vi "pessimize_error.vi"(8 "End transform offset":dbl[](array[numeric])=[0.0, 0.0, 0.0, 0.0, 0.0, 0.0] format="%#.3f", 9 "stop":refnum<vi>, 10 "Point selector":T7 {"Light number" min=0 max=5}, 11 "Override in":T6) -> ()   [LabVIEW 2013]
uses:
  calibration/point_selector.ctl
  ui_override_opts.ctl
  pessimize_objective_fun_info.ctl
  pressimize_state.ctl
  <vilib>/Utility/file.llb/Write To Spreadsheet File (DBL).vi
  <vilib>/Analysis/Matrix/Datatypes/RealMatrix.ctl
  <vilib>/Analysis/Matrix/NI_Matrix.lvlib
  <vilib>/gmath/NumericalOptimization/stopping criteria.ctl
  <vilib>/gmath/NI_Gmath.lvlib
panel:
  in  "Save":bool
  in  "Save file":path
  out "Trials":T1 format="%#_3p"
  in  "Random trials":i32=1
  out "Error vector":T1 format="%#_3p"
  out "Pose bias":T1 format="%#_3p"
  out "f(X) max":dbl format="%#_3p"
  in  "Random":bool
  in  "Last out":bool
  in  "GD gain":dbl=0.3
  in  "dX":T1=[[0.2, 1.0]]
  in  "Method":T2(ring)
  in  "Local stop":bool
  in  "Trace length":dbl=0.2
  in  "Moment":dbl=50.0
  in  "XY plots":cluster{"X":T3, "Y":T3}[](array[cluster])=[{"X"=enum."X", "Y"=enum."Y"}, {"X"=enum."X", "Y"=enum."Z"}, {"X"=enum."Rx", "Y"=enum."Ry"}, {"X"=enum."Rx", "Y"=enum."Rz"}]
  out "XY Graph":T4(graph)
  out "Function calls":i32 caption="Iterations"
  out "Function value":dbl[](graph)
  in  "Running":bool
  in  "Start point":T1 format="%#_3p"
  in  "Workspace bounds":T1=[[-15.0, -15.0, -15.0, -20.0, -20.0, -10.0], [15.0, 15.0, 15.0, 10.0, 20.0, 10.0]]
  in  "Optimization status":T1 format="%#_3p"
  in  "Scaling":T1=[[1.0, 0.2], [0.1, 1.0], [0.1, 0.1]]
  in  "Error criterion":enum16{"Translation", "Orientation", "Moment"}(ring)
  out "X at maximum":T1 format="%#_3p"
  in  "stopping criteria":T5={"function tolerance"=1.0, "parameter tolerance"=0.1, "max iterations"=100, "max function calls"=1000, "gradient tolerance"=0.01, "max time (sec)"=-1.0}
  # "--------XYZ--------      ---------Rxyz---------     --------eXYZ---------      --------eRxyz-------      eFun"
  # "XYZ"
  # "R"
  # "Min"
  # "Max"
  # "X"
  # "Y"
  # "Z"
  # "Rx"
  # "Ry"
  # "Rz"
  # "--------XYZ--------      ---------Rxyz---------     --------eXYZ---------      --------eRxyz-------      eFun       ------gradXYZ------      ------gradRxyz------"
  # "XYZ error"
  # "R error"
  # "Tolerance"
  # "Trans"
  # "Orient"
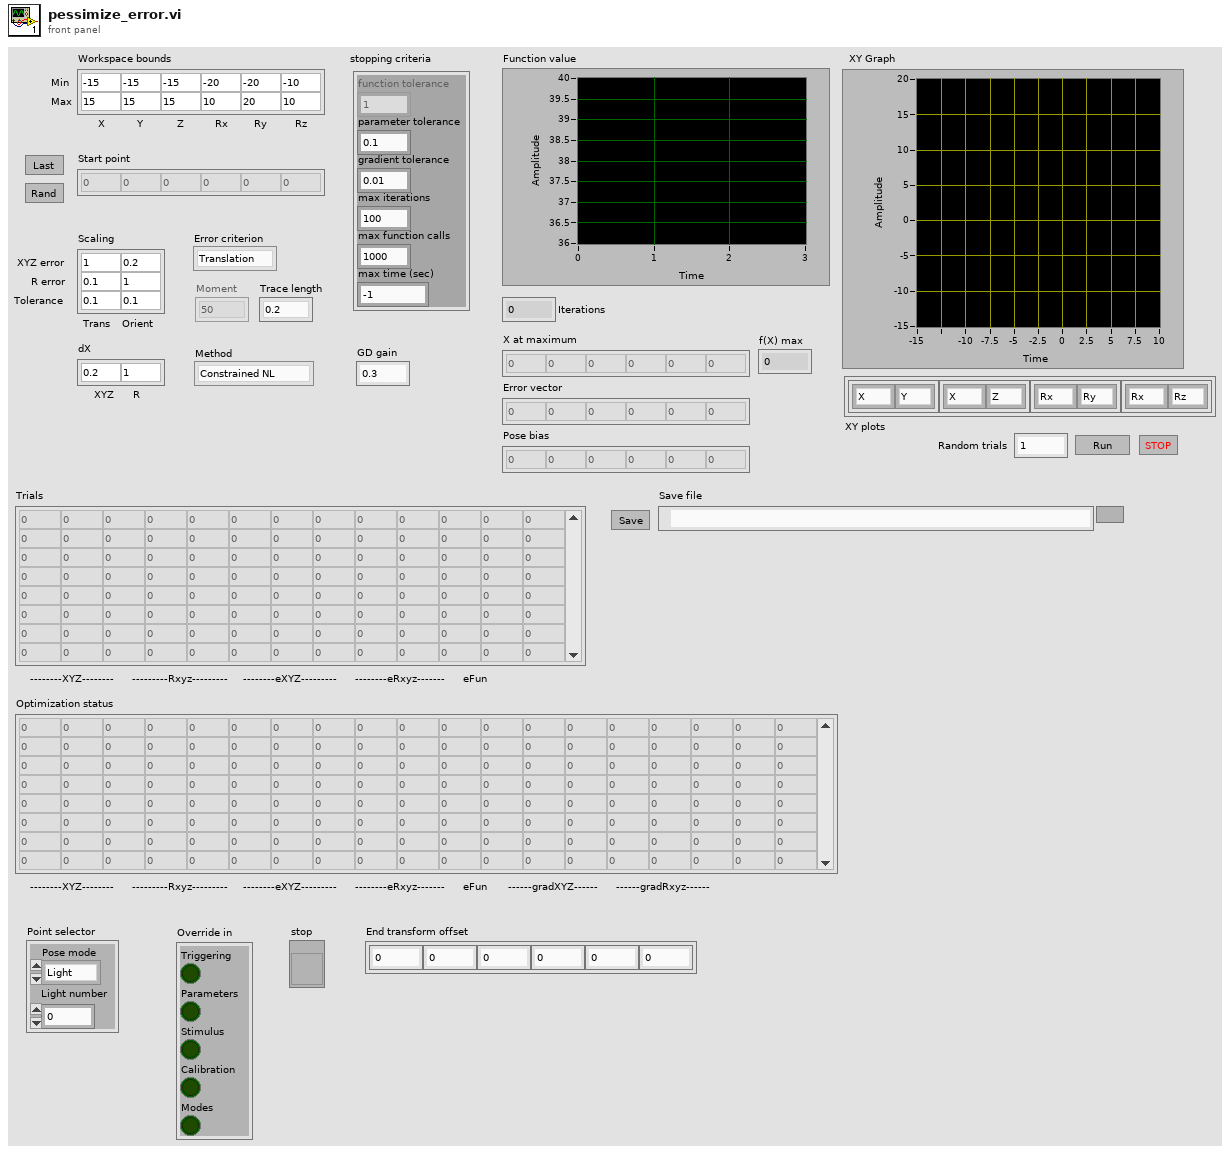
[diagram p1: front panel]
types:
  T1 = typedef "NI_Matrix.lvlib/RealMatrix.ctl" = dbl[][]
  T2 = enum16{"Constrained NL", "Simplex", "Gradient descent"}
  T3 = typedef "pressimize_state.ctl" = enum16{"X", "Y", "Z", "Rx", "Ry", "Rz", "eX", "eY", "eZ", "eRx", "eRy", "eRz", "eFun", "gX", "gY", "gZ", "gRx", "gRy", "gRz"}
  T4 = cluster{"Optimization status":dbl[], "Optimization status":dbl[]}[]
  T5 = typedef "NI_Gmath.lvlib/stopping criteria.ctl" = cluster{"function tolerance":dbl, "parameter tolerance":dbl, "max iterations":i32, "max function calls":i32, "gradient tolerance":dbl, "max time (sec)":dbl}
  T6 = typedef "ui_override_opts.ctl" = cluster{"Triggering":bool, "Parameters":bool, "Stimulus":bool, "Calibration":bool, "Modes":bool}
  T7 = typedef "point_selector.ctl" = cluster{"Pose mode":enum16{"Light", "Handle", "Output"}, "Light number":i32}
  T8 = enum8{"Enabled", "Disabled", "Disabled and Grayed Out"}
  T9 = typedef "pessimize_objective_fun_info.ctl" = cluster{"Error criterion":enum16{"Translation", "Orientation", "Moment"}, "Scale factors":dbl[], "Gradient increment":dbl[], "Pose bias":dbl[], "Extra end transform":dbl[], "Point selector":T7, "Trace length":dbl, "Override in":T6, "Optimization status":refnum<vi>, "stop":refnum<vi>}
  T10 = cluster{"Method":enum16{"Constrained NL", "Simplex", "Gradient descent"}, "Scaling":T1, "Moment":dbl, "dX":T1, "stopping criteria":T5, "Workspace bounds":T1, "GD gain":dbl}
  T11 = cluster{"Optimization status":dbl[], "Optimization status":dbl[]}
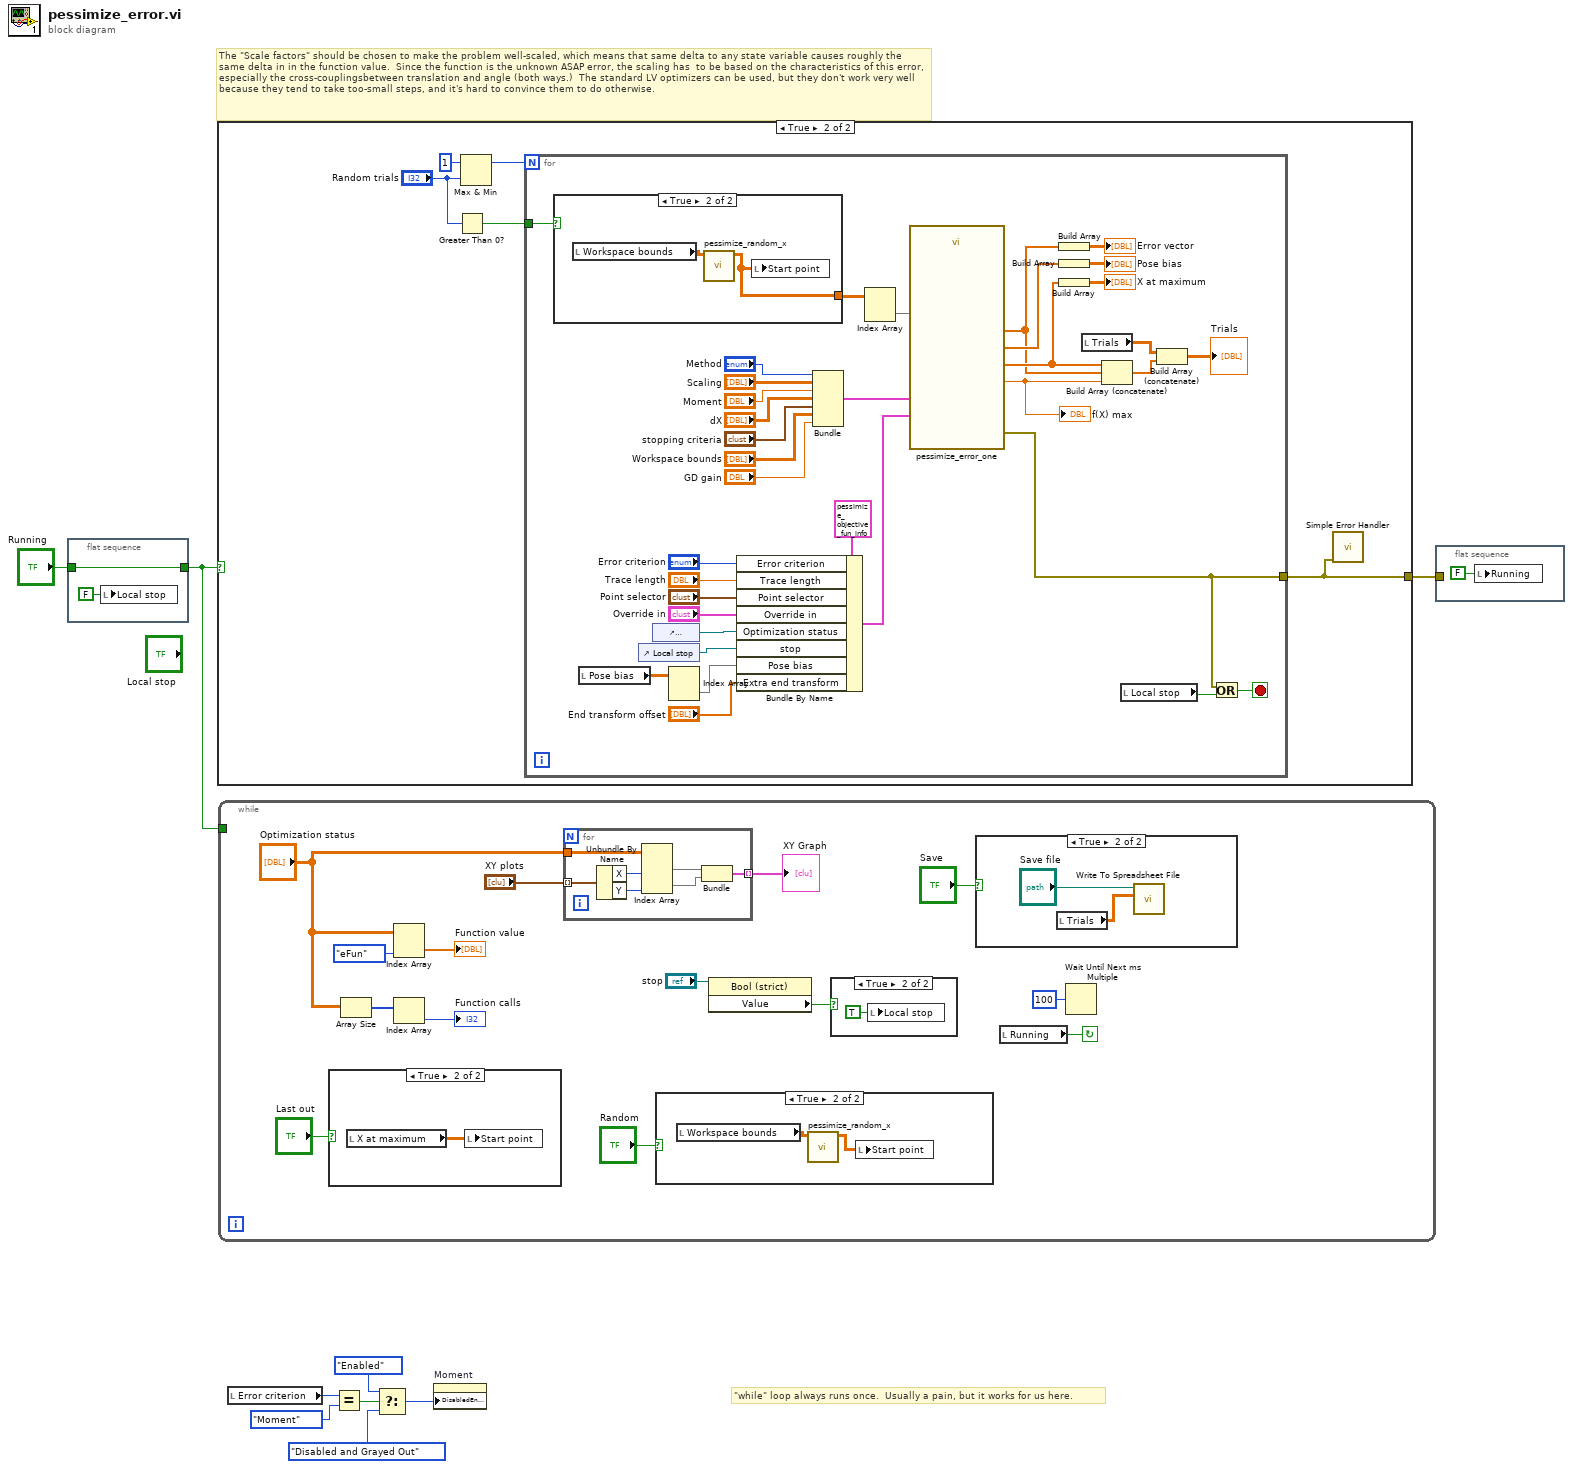
[diagram p0: block diagram]
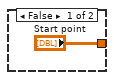
[diagram p7: hidden frame]
diagram:
  # "The \"Scale factors\" should be chosen to make the problem well-scaled, which means that same delta to any state variable causes roughly the same delta in in the function value.  Since the function is the unknown ASAP error, the scaling has  to be based on the characteristics of this error, especially the cross-couplingsbetween translation and angle (both ways.)  The standard LV optimizers can be used, but they don't work very well because they tend to take too-small steps, and it's hard to convince them to do otherwise."
  # "\"while\" loop always runs once.  Usually a pain, but it works for us here."
  n1 = flat-sequence {
    tunnel: [w10] -> w2
    tunnel: "Running" -> [w10]
    frame #0 {
      n2 = local write "Local stop"(FALSE ("Local stop")) -> ()
    }
  }
  n3 = case shown="True" w2 {
    tunnel: [_ w16] -> w9
    frame False {
    }
    frame True {
      n4 = Greater Than 0?(x="Random trials") -> (x > 0?=w12:bool)
      n5 = Max & Min(x=1, y="Random trials") -> (max(x,y)=w14:i32)  [unwired: 1 out]
      n6 = for {
        N: w14 -> [_]
        tunnel: [w19] -> w16
        tunnel: w12 -> [w21]
        stop <- w18 stop-if-true
        n7 = case shown="True" w21 {
          tunnel: ["Start point" w53] -> w23
          frame False {
          }
          frame True {
            n8 = local read "Workspace bounds"() -> (w54:T1)
            n9 = call "pessimize_random_x.vi"("Workspace bounds"=w54) -> ("Array"=w53:dbl[][])  [unwired: 10 in]
            n10 = local write "Start point"(w53) -> ()
          }
        }
        n11 = local read "Pose bias"() -> (w44:T1)
        n12 = control-ref of="Local stop"() -> (w45:refnum<vi>)
        n13 = control-ref of="Optimization status"() -> (w48:refnum<vi>)
        n14 = Index Array(array=w44) -> (element=w43:dbl[])  [unwired: 2 in]
        n15 = Bundle By Name(cluster=T9 {"Error criterion"=enum."Translation", "Scale factors"=[], "Gradient increment"=[], "Pose bias"=[], "Extra end transform"=[], "Point selector"={"Pose mode"=enum."Light", "Light number"=0}, "Trace length"=0.0, "Override in"={"Triggering"=FALSE, "Parameters"=FALSE, "Stimulus"=FALSE, "Calibration"=FALSE, "Modes"=FALSE}, "Optimization status"=refnum, "stop"=refnum} ("Pessimize fun info"), "Error criterion"="Error criterion", "Trace length"="Trace length", "Point selector"="Point selector", "Override in"="Override in", "Optimization status"=w48, "stop"=w45, "Pose bias"=w43, "Extra end transform"="End transform offset") -> (w42:T9)
        n16 = Bundle("Method"="Method", "Scaling"="Scaling", "Moment"="Moment", "dX"="dX", "stopping criteria"="stopping criteria", "Workspace bounds"="Workspace bounds", "GD gain"="GD gain") -> (w34:T10)  [unwired: 1 in]
        n17 = Index Array(array=w23) -> (element=w22:dbl[])  [unwired: 2 in]
        n18 = call "pessimize_error_one.vi"("Parameters"=w34, "Start point"=w22, "Pessimize fun info"=w42) -> ("Pose bias"=w30:dbl[], "Error vector"=w28:dbl[], "f(X)"=w27:dbl, "X at maximum"=w29:dbl[], "error out"=w19:errorcluster)  [unwired: 8 in]
        "f(X) max" <- w27
        n19 = Build Array(w28) -> (→"Error vector":dbl[][])
        n20 = Build Array(w30) -> (→"Pose bias":dbl[][])
        n21 = Build Array(w29) -> (→"X at maximum":dbl[][])
        n22 = local read "Trials"() -> (w26:T1)
        n23 = Build Array (concatenate)(w29, w28, w27) -> (w25:dbl[])
        n24 = local read "Local stop"() -> (w20:bool)
        n25 = Build Array (concatenate)(w26, w25) -> (→"Trials":T1)
        n26 = Or(x=w19, y=w20) -> (x .or. y?=w18:bool)
      }
      n27 = call <vilib>:"Simple Error Handler.vi"("error in (no error)"=w16) -> ()  [unwired: 4 in, 5 out]
    }
  }
  n28 = while {
    tunnel: w2 -> [_]
    stop <- w68 continue-if-true
    n29 = case shown="True" "Last out" {
      frame False {
      }
      frame True {
        n30 = local read "X at maximum"() -> (w73:T1)
        n31 = local write "Start point"(w73) -> ()
      }
    }
    n32 = Array Size(array="Optimization status") -> (size(s)=w64:i32[])
    n33 = Index Array(array="Optimization status", index (col)=pressimize_state."eFun" ("Pessimize state")) -> (element=→"Function value":dbl[])  [unwired: 1 in]
    n34 = Index Array(array=w64) -> (element=→"Function calls":i32)  [unwired: 1 in]
    n35 = for {
      tunnel: "XY plots" -> [w80] mode=indexing
      tunnel: "Optimization status" -> [w81]
      tunnel: [w75] -> w62 mode=indexing
      n36 = Unbundle By Name(w80) -> ("X"=w79:T3, "Y"=w78:T3)
      n37 = Index Array(array=w81, index (col) #1=w79, index (col) #2=w78) -> (element #1=w77:dbl[], element #2=w76:dbl[])  [unwired: 2 in]
      n38 = Bundle("Optimization status"=w77, "Optimization status"=w76) -> (w75:T11)  [unwired: 1 in]
    }
    "XY Graph" <- w62
    n39 = case shown="True" "Random" {
      frame False {
      }
      frame True {
        n40 = local read "Workspace bounds"() -> (w72:T1)
        n41 = call "pessimize_random_x.vi"("Workspace bounds"=w72) -> ("Array"=w71:dbl[][])  [unwired: 10 in]
        n42 = local write "Start point"(w71) -> ()
      }
    }
    n43 = property class="Bool (strict)"(reference="stop") -> ("Value"=w60:bool)  [unwired: 1 in, 2 out]
    n44 = case shown="True" w60 {
      frame False {
      }
      frame True {
        n45 = local write "Local stop"(TRUE ("Local stop")) -> ()
      }
    }
    n46 = case shown="True" "Save" {
      frame False {
      }
      frame True {
        n47 = local read "Trials"() -> (w69:T1)
        n48 = call-poly <vilib>:"Write To Spreadsheet File.vi"("2D data"=w69, "file path (dialog if empty)"="Save file") -> ()  [unwired: 6 in, 1 out]
      }
    }
    n49 = local read "Running"() -> (w68:bool)
    n50 = Wait Until Next ms Multiple(millisecond multiple=u32 100) -> ()  [unwired: 1 out]
  }
  n51 = local read "Error criterion"() -> (w8:enum16{"Translation", "Orientation", "Moment"})
  n52 = Equal?(x=w8, y=enum16{"Translation", "Orientation", "Moment"}."Moment" ("Error criterion")) -> (x = y?=w6:bool)
  n53 = Select(t=T8."Enabled" ("Disabled"), s=w6, f=T8."Disabled and Grayed Out" ("Disabled")) -> (s? t:f=w3:T8)
  n54 = property on="Moment" class="DigNum (strict)"("DisabledEnum"=w3) -> ()  [unwired: 2 in, 2 out]
  n55 = flat-sequence {
    tunnel: w9 -> [_]
    frame #0 {
      n56 = local write "Running"(FALSE ("Running")) -> ()
    }
  }
